vi "NI 9411 TASK.vi"(6 "divisor":u32=4, 8 "error in":errorcluster, 9 "CI.Freq.Term":tag="/CDRMod7/PFI3", 11 "MODULE NAME":string="cDAQ_NICOTRAMod5/ctr0") -> (0 "error out":errorcluster, 3 "task out":refnum<k21>)   [LabVIEW 2019]
uses:
  <vilib>/DAQmx/create/channels.llb/DAQmx Create Channel (CI-Frequency).vi
  <resource>/objmgr/daqmx.rc
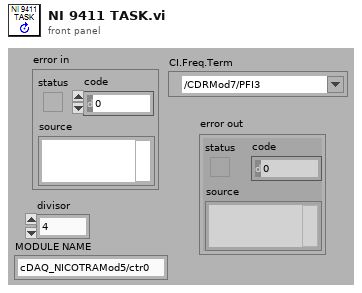
[diagram p1: front panel]
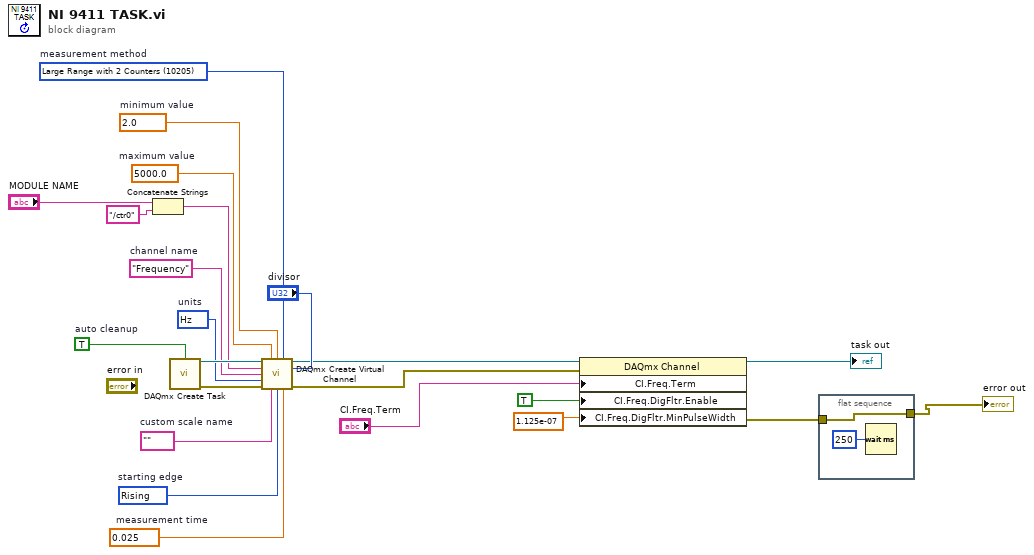
[diagram p0: block diagram]
diagram:
  w10 = tag ""  # custom scale name
  w11 = 10280 items=["Rising"=10280, "Falling"=10171]  # starting edge
  w15 = 10373 items=["Hz"=10373, "Ticks"=10304, "From Custom Scale"=10065]  # units
  w16 = 0.025  # measurement time
  w6 = 10205 items=["Low Frequency with 1 Counter"=10105, "High Frequency with 2 Counters"=10157, "Large Range with 2 Counters"=10205]  # measurement method
  w18 = "Frequency"  # channel name
  w19 = 2.0  # minimum value
  w20 = 5000.0  # maximum value
  w22 = TRUE  # auto cleanup
  n1 = Concatenate Strings("MODULE NAME", "/ctr0" ("string")) -> (w5:string)
  n2 = call <vilib>:"DAQmx Create Task.vi"("auto cleanup"=w22) -> ("task out"=w21:refnum<k21>, "error out"=w23:errorcluster)  [unwired: 13 in]
  n3 = call-poly <vilib>:"DAQmx Create Virtual Channel.vi"("task in"=w21, "maximum value"=w20, "minimum value"=w19, "measurement method"=w6, "counter"=w5, "divisor"="divisor", "name to assign"=w18, "units"=w15, "error in"=w23, "custom scale name"=w10, "starting edge"=w11, "measurement time"=w16) -> ("task out"=w12:refnum<k21>, "error out"=w9:errorcluster)  [unwired: 2 in]
  n4 = property class="DAQmx Channel"(reference=w12, error in=w9, "CI.Freq.Term"="CI.Freq.Term", "CI.Freq.DigFltr.Enable"=TRUE ("DI.DigFltr.Enable"), "CI.Freq.DigFltr.MinPulseWidth"=1.125e-07 ("DI.DigFltr.MinPulseWidth")) -> (reference out=→"task out":refnum<k21>, error out=w8:errorcluster)
  n5 = flat-sequence {
    tunnel: [w24] -> w7
    tunnel: w8 -> [w24]
    frame #0 {
      n6 = Wait (ms)(milliseconds to wait=u32 250) -> ()  [unwired: 1 out]
    }
  }
  "error out" <- w7
